vi "FMDLFilePath.vi"(0 "Extra comment":string, 1 "Repetition Number":u32, 4 "Include seconds string?":bool=TRUE, 5 "Include Year Month string?":bool=TRUE, 6 "Experiment number":u32=1, 7 "Experiment Name":string, 8 "Experiment Type":string, 9 "Data folder":path) -> (2 "date/time string":string, 3 "Unique Filepath":path)   [LabVIEW 2018]
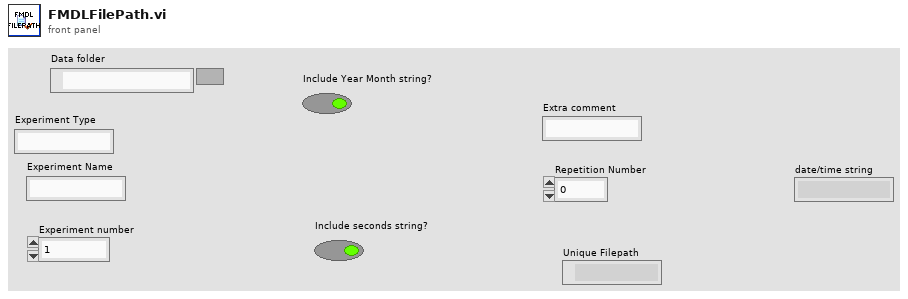
[diagram p1: front panel]
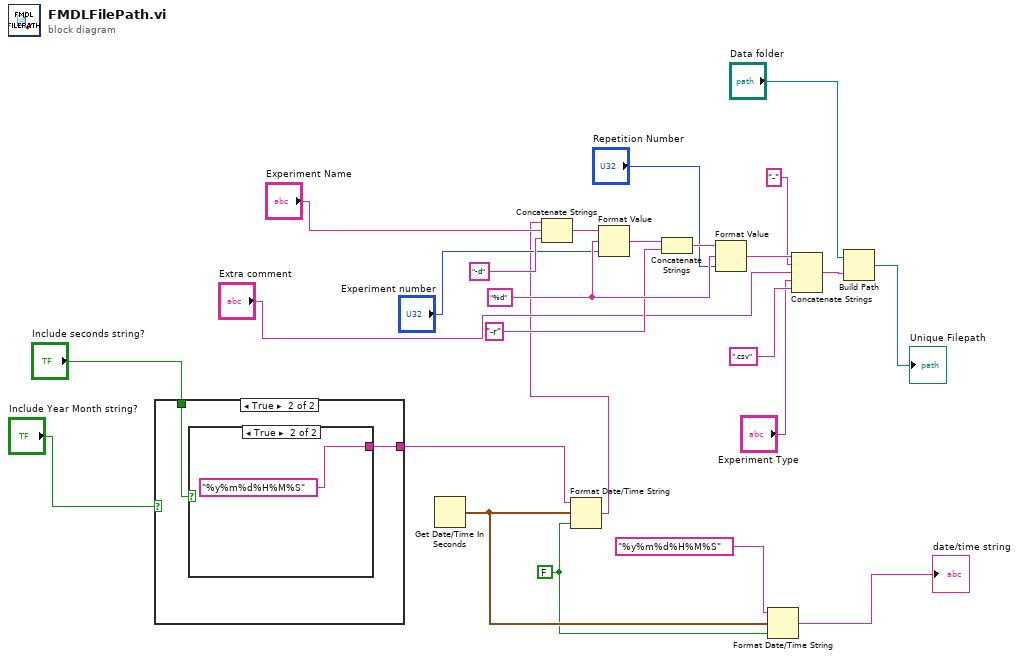
[diagram p0: block diagram]
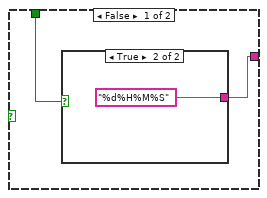
[diagram p2: hidden frame]
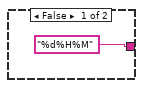
[diagram p3: hidden frame]
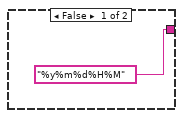
[diagram p4: hidden frame]
diagram:
  w2 = FALSE ("UTC format")
  w23 = "%d"
  n1 = case shown="True" "Include Year Month string?" {
    tunnel: [w26 w31] -> w15
    tunnel: "Include seconds string?" -> [w27 w30]
    frame False {
      n2 = case shown="True" w27 {
        tunnel: ["%d%H%M" ("time format string (%c)") "%d%H%M%S" ("time format string (%c)")] -> w26
        frame False {
        }
        frame True {
        }
      }
    }
    frame True {
      n3 = case shown="True" w30 {
        tunnel: ["%y%m%d%H%M" ("time format string (%c)") "%y%m%d%H%M%S" ("time format string (%c)")] -> w31
        frame False {
        }
        frame True {
        }
      }
    }
  }
  n4 = Get Date/Time In Seconds() -> (seconds since 1Jan1904=w3:timestamp)
  n5 = Format Date/Time String(time format string (%c)=w15, seconds (now)=w3, UTC format=w2) -> (date/time string=w5:string)
  n6 = Concatenate Strings(w5, "Experiment Name", "-d") -> (w24:string)
  n7 = Format Value(string ("")=w24, format string=w23, value (0)="Experiment number") -> (output string=w22:string)
  n8 = Concatenate Strings(w22, "-r") -> (w20:string)
  n9 = Format Value(string ("")=w20, format string=w23, value (0)="Repetition Number") -> (output string=w19:string)
  n10 = Format Date/Time String(time format string (%c)="%y%m%d%H%M%S", seconds (now)=w3, UTC format=w2) -> (date/time string=→"date/time string":string)
  n11 = Concatenate Strings(w19, "-", "Extra comment", "Experiment Type", ".csv") -> (w18:string)
  n12 = Build Path(base path="Data folder", name or relative path=w18) -> (appended path=→"Unique Filepath":path)
